vi "초음파 센서.vi"() -> ()   [LabVIEW 2010]
uses:
  <vilib>/NXT/Block Support/NXT_InputPort.ctl
  <vilib>/NXT/Dual Mode Library/Sound/Tone.vi
panel:
  out "Waveform Chart":i16(graph)
  out "Distance (cm)":i16
  in  "Port (Port 4)":T1=3 items=["Port 1", "Port 2", "Port 3", "Port 4"]
  in  "stop":bool
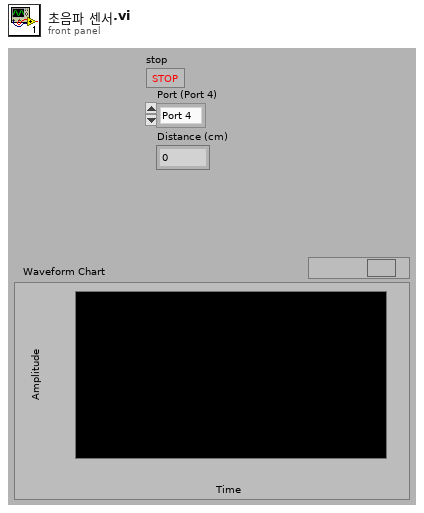
[diagram p1: front panel]
types:
  T1 = typedef "NXT_InputPort.ctl" = u8
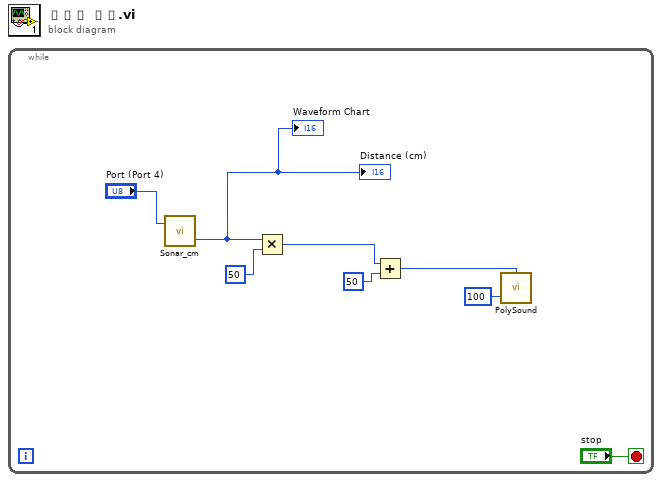
[diagram p0: block diagram]
diagram:
  n1 = while {
    stop <- "stop" stop-if-true
    n2 = call <vilib>:"Sonar_cm.vi"("Port (Port 4)"="Port (Port 4)") -> ("Distance (cm)"=w1:i16)  [unwired: 2 in, 1 out]
    "Distance (cm)" <- w1
    "Waveform Chart" <- w1
    n3 = Multiply(x=w1, y=i16 50) -> (x*y=w8:i16)
    n4 = Add(x=w8, y=i16 50) -> (x+y=w7:i16)
    n5 = call-poly <vilib>:"PolySound.vi"("Duration (500 ms)"=u16 100, "Tone (440 Hz)"=w7) -> ()  [unwired: 2 in, 1 out]
  }
